vi "Update Graph Axis Names.vi"(0 "Graph":refnum<vi>, 5 "Axis Names":string[](array[string])) -> ()   [LabVIEW 2019]
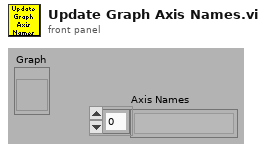
[diagram p1: front panel]
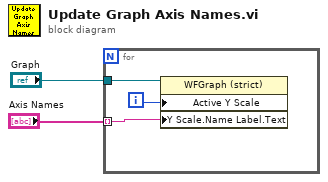
[diagram p0: block diagram]
diagram:
  n1 = for {
    tunnel: "Graph" -> [w5]
    tunnel: "Axis Names" -> [w3] mode=indexing
    i -> [w4]
    n2 = property class="WFGraph (strict)"(reference=w5, "Active Y Scale"=w4, "Y Scale.Name Label.Text"=w3) -> ()  [unwired: 1 in, 2 out]
  }
